vi "1Darray_mean_sub.vi"(1 "1D array":dbl[](array[numeric])) -> (0 "Mean":dbl)   [LabVIEW 2021]
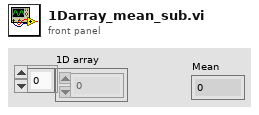
[diagram p1: front panel]
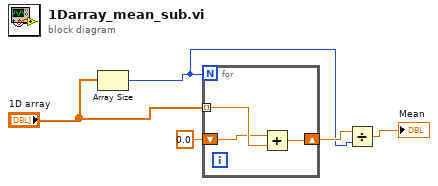
[diagram p0: block diagram]
diagram:
  n1 = Array Size(array="1D array") -> (size(s)=w1:i32)
  n2 = for {
    N: w1 -> [_]
    tunnel: "1D array" -> [w8] mode=indexing
    shift-right: [w7] -> w2
    shift-left: 0.0 -> [w6]
    n3 = Add(x=w6, y=w8) -> (x+y=w7:dbl)
  }
  n4 = Divide(x=w2, y=w1) -> (x/y=→"Mean":dbl)
